vi "INSERT.vi"(6 "Time Stamp":timestamp, 8 "error in":errorcluster, 9 "Data":variant, 10 "Path(s)":variant, 11 "Data.PG in":refnum<class "Data.PGSQL.lvclass">) -> (0 "error out":errorcluster, 2 "Wrote to DB?":bool, 3 "Data.PG out":refnum<class "Data.PGSQL.lvclass">)   [LabVIEW 2013, in "Data.PGSQL.lvclass"]
uses:
  Data.PGSQL.lvclass
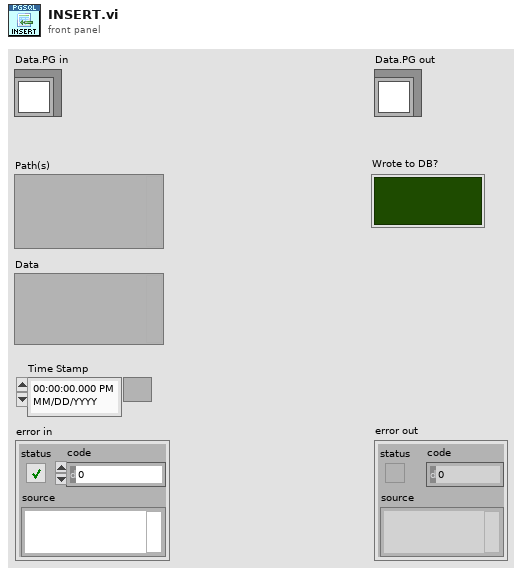
[diagram p1: front panel]
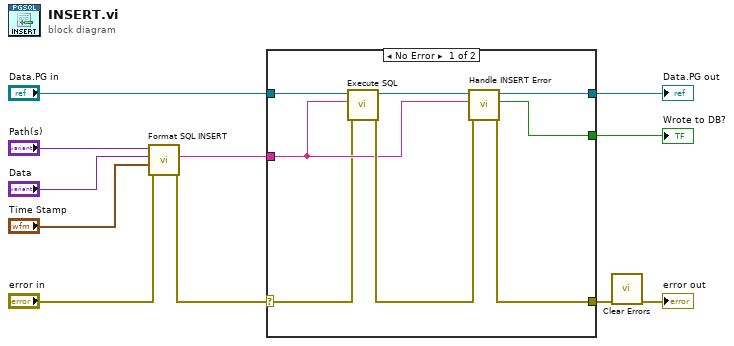
[diagram p0: block diagram]
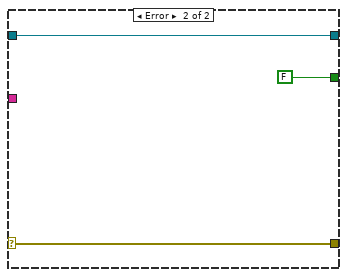
[diagram p2: hidden frame]
diagram:
  n1 = call "Format SQL INSERT.vi"("error in"="error in", "Time Stamp"="Time Stamp", "Data"="Data", "Path(s)"="Path(s)") -> ("error out"=w3:errorcluster, "Formatted Insert"=w6:string)  [unwired: 6 in]
  n2 = case shown="No Error" w3 {
    selector: w3 -> [w13 w20]
    tunnel: [w12 w20] -> w11
    tunnel: "Data.PG in" -> [w17 w22]
    tunnel: [w19 w22] -> w9
    tunnel: [w18 FALSE] -> w8
    tunnel: w6 -> [w14 _]
    frame No Error {
      n3 = call "Execute SQL.vi"("error in"=w13, "SQL"=w14, "Data.PG"=w17) -> ("error out"=w15:errorcluster, "Data.PG out"=w16:refnum<class "Data.PGSQL.lvclass">)  [unwired: 6 in, 1 out]
      n4 = call "Handle INSERT Error.vi"("error in (no error)"=w15, "SQL"=w14, "Database.PG"=w16) -> ("error out"=w12:errorcluster, "Wrote to DB?"=w18:bool, "Database.PG out"=w19:refnum<class "Data.PGSQL.lvclass">)  [unwired: 6 in]
    }
    frame Error {
    }
  }
  "Data.PG out" <- w9
  "Wrote to DB?" <- w8
  n5 = call <vilib>:"Clear Errors.vi"("error in (no error)"=w11) -> ("error out"=→"error out":errorcluster)  [unwired: 5 in, 1 out]
